vi "IFFT_design.vi"(7 "index":i32, 8 "data_len":i32, 9 "dl":i32, 10 "din":cdb[](array[numeric]), 11 "Sdl":i32) -> (2 "dout":cdb[](array[numeric]))   [LabVIEW 2010]
uses:
  <vilib>/imath/engines/lvmath2/RunTimeEngine/ErrorHandling/NIMS_Finalize Error.vi
  <vilib>/imath/engines/lvmath2/RunTimeEngine/NodeEndStatement/NIMS_NodeEndStatement_Output.vi
  <instcachedir>/0/NIMS_NodeEndStatement_Output_53EC0D466D134D7ABD903AC30B43404B.lvgen/NIMS_NodeEndStatement_Output_53EC0D466D134D7ABD903AC30B43404B_000.vi
  <vilib>/imath/engines/lvmath2/RunTimeEngine/BuiltInFunctions/zeros/NIMS_V=zeros(I32,I32).vi
  <vilib>/imathl/engines/lvmath/Functions/Error Handling/Create Error.vi
  <vilib>/imath/engines/lvmath2/RunTimeEngine/RangeToken/NIMS_Range_R2 - Float.vi
  <instcachedir>/0/NIMS_Range_R2 - Float_B141A161314947C2A0872DED502D7279.lvgen/NIMS_Range_R2 - Float_B141A161314947C2A0872DED502D7279_000.vi
  <vilib>/imath/engines/lvmath2/RunTimeEngine/CommandStatement/MC_CommandStatement_break.vi
  <vilib>/imath/engines/lvmath2/RunTimeEngine/RangeToken/NIMS_Range.vi
  <instcachedir>/0/NIMS_Range_1C63927E4E474DADACDA97C3F2261A11.lvgen/NIMS_Range_1C63927E4E474DADACDA97C3F2261A11_001.vi
  <vilib>/imath/engines/lvmath2/RunTimeEngine/ReplaceToken/NIMS_Replace - Check(_) Linear.vi
  <instcachedir>/0/NIMS_Replace - Check(_) Linear_D531E313C4004E3DB8F0EA3CE86AE758.lvgen/NIMS_Replace - Check(_) Linear_D531E313C4004E3DB8F0EA3CE86AE758_007.vi
  <vilib>/imath/engines/lvmath2/RunTimeEngine/VariableToken/Read/NIMS_Get Elements - RV(_) - Check(_).vi
  <instcachedir>/0/NIMS_Get Elements - RV(_) - Check(_)_260A45C9C4AF472A8F32F86A1BEF7DEE.lvgen/NIMS_Get Elements - RV(_) - Check(_)_260A45C9C4AF472A8F32F86A1BEF7DEE_001.vi
  <vilib>/imath/engines/lvmath2/RunTimeEngine/BuiltInFunctions/ifft/NIMS_ifft(CV).vi
  <vilib>/imath/engines/lvmath2/RunTimeEngine/ReplaceToken/NIMS_Replace - Size Check _(_)=VorM.vi
  <instcachedir>/0/NIMS_Replace - Size Check _(_)=VorM_4228B35EE910471DB74F3866D9D09B95.lvgen/NIMS_Replace - Size Check _(_)=VorM_4228B35EE910471DB74F3866D9D09B95_007.vi
  <vilib>/imath/engines/lvmath2/RunTimeEngine/ReplaceToken/NIMS_Replace - Assignment Check _(_)=VorM.vi
  <instcachedir>/0/NIMS_Replace - Assignment Check _(_)=VorM_C130F3B8B64B4DD7B9359A2D3A035D18.lvgen/NIMS_Replace - Assignment Check _(_)=VorM_C130F3B8B64B4DD7B9359A2D3A035D18_007.vi
  <vilib>/imath/engines/lvmath2/RunTimeEngine/ErrorHandling/NIMS_Create Error From Enums.vi
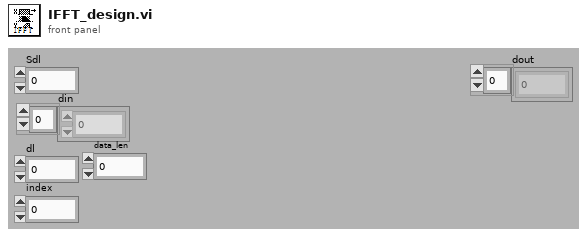
[diagram p1: front panel]
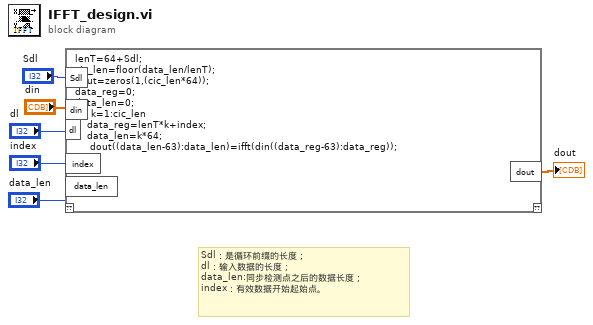
[diagram p0: block diagram]
diagram:
  # "Sdl：是循环前缀的长度；\ndl：输入数据的长度；\ndata_len:同步检测点之后的数据长度；\nindex：有效数据开始起始点。"
  n1 = mathscript code="lenT=64+Sdl;\ncic_len=floor(data_len/lenT);\ndout=zeros(1,(cic_len*64));\ndata_reg=0;\ndata_len=0;\nfor k=1:cic_len\n    data_reg=lenT*k+index;\n    data_len=k*64;\n     dout((data_len-63):data_len)=ifft(din((data_reg-63):data_reg));\nend"("din"="din", "dl"="dl", "index"="index", "data_len"="data_len", "Sdl"="Sdl") -> ("dout"=→"dout":cdb[])  [unwired: 1 in, 1 out]
